vi "publish -- read.vi"(8 "request event":refnum<user-event>, 9 "recieve event":refnum<user-event>) -> (1 "recieve event OUT":refnum<user-event>)   [LabVIEW 2018]
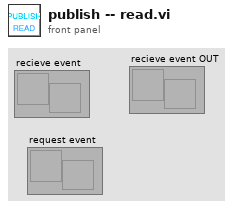
[diagram p1: front panel]
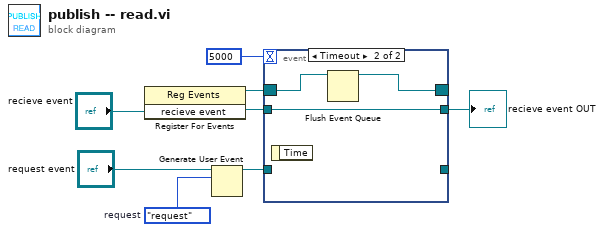
[diagram p0: block diagram]
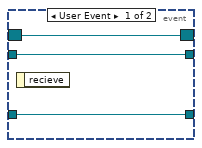
[diagram p2: hidden frame]
diagram:
  w7 = enum16{"request"}."request"  # request
  n1 = register-events("recieve event") -> (reference out=w4:refnum<event-registration>)  [unwired: 2 in, 1 out]
  n2 = Generate User Event(user event="request event", event data cluster=w7) -> (user event out=w5:refnum<user-event>)  [unwired: 2 in, 1 out]
  n3 = event shown="[1] Timeout" {
    selector: w4 -> [w9 w13]
    dyn-events: [w9 w12] -> _
    timeout: 5000 -> [_ _]
    tunnel: [w10 _] -> _
    tunnel: w5 -> [w10 _]
    tunnel: [w8 w11] -> w2
    tunnel: "recieve event" -> [w8 w11]
    event User Event {
      n4 = event-data() -> ()  [unwired: 1 in, 1 out]
    }
    event Timeout {
      n5 = event-data() -> ()  [unwired: 1 in, 1 out]
      n6 = Flush Event Queue(0:w13) -> (8:w12:refnum<event-registration>)  [unwired: 5 in, 2 out]
    }
  }
  "recieve event OUT" <- w2
